vi "Test Replace Configuration Table By ID.vi"() -> ()   [LabVIEW 2017]
uses:
  user.lib/NEVSTOP-Programming-Palette/Configuration/ClusterCfgTable/_instance/_Replace Configuration Table By ID(Element).vi
  user.lib/NEVSTOP-Programming-Palette/Configuration/ClusterCfgTable/_instance/_Replace Configuration Table By ID(Array).vi
panel:
  in  "Array 3":string[][](array[string])=[["11", "IDa", "xx", "gg"], ["1222", "IDb", "bb", "cc"]]
  in  "Array 2":string[](array[string])=["11", "IDa", "xx", "gg"]
  in  "Array":string[][](array[string])=[["1", "IDa", "x", "g"], ["#", "IDb", "y", "f"], ["2", "IDc", "z", "e"], ["3", "IDd", "a", "d"], ["4", "IDb", "b", "c"]]
  out "Table out 2":string[][](array[string])=[["11", "IDa", "xx", "gg"], ["#", "IDb", "y", "f"], ["2", "IDc", "z", "e"], ["3", "IDd", "a", "d"], ["1222", "IDb", "bb", "cc"]]
  out "Table out":string[][](array[string])=[["11", "IDa", "xx", "gg"], ["#", "IDb", "y", "f"], ["2", "IDc", "z", "e"], ["3", "IDd", "a", "d"], ["4", "IDb", "b", "c"]]
  # "ID"
  # "ID"
  # "ID"
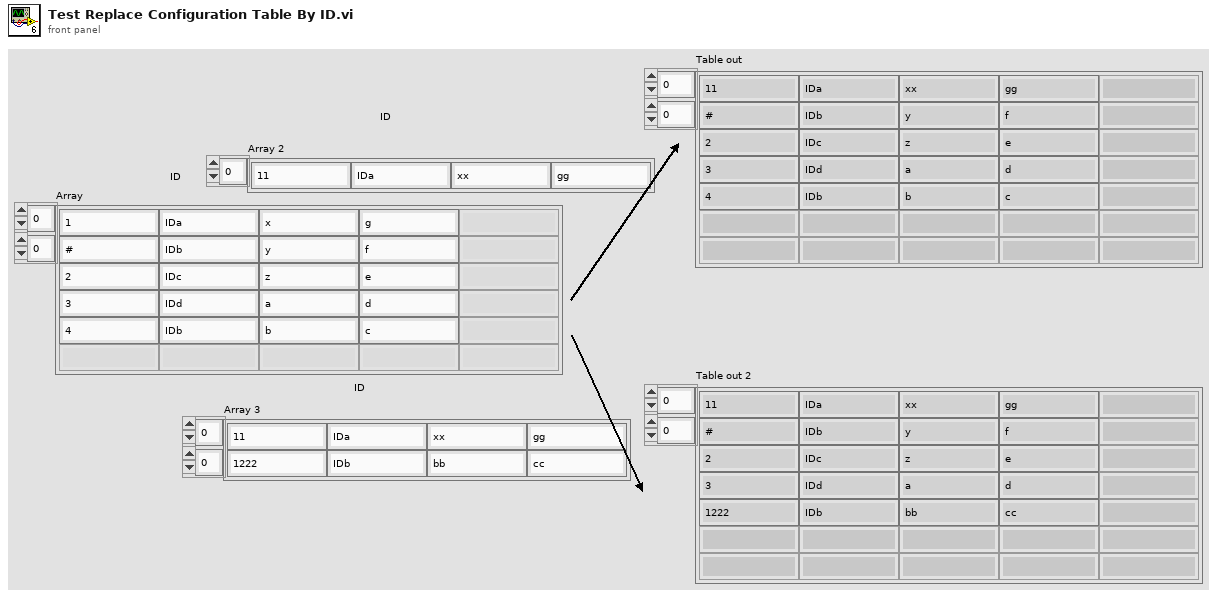
[diagram p1: front panel]
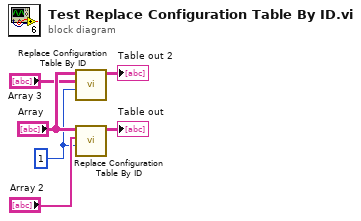
[diagram p0: block diagram]
diagram:
  w1 = 1 ("ID Col")
  n1 = call-poly "Replace Configuration Table By ID.vi"("ID Col"=w1, "New Line"="Array 3", "Table in"="Array") -> ("Table out"=→"Table out 2":string[][])  [unwired: 7 in, 1 out]
  n2 = call-poly "Replace Configuration Table By ID.vi"("ID Col"=w1, "New Line"="Array 2", "Table in"="Array") -> ("Table out"=→"Table out":string[][])  [unwired: 7 in, 1 out]
